vi "Video Processing.vi"() -> ()   [LabVIEW 2014]
uses:
  Global.vi
panel:
  out "Number of Particles before":i32
  out "Processed Image":T1(plugin-control)
  out "Number of Particles after":i32
  out "Original":T1(plugin-control)
  in  "Number of Erosion":i32=30
  out "x-y":u32=48
  out "Read Video":errorcluster
  in  "stop video":bool
  in  "milliseconds to wait":u32
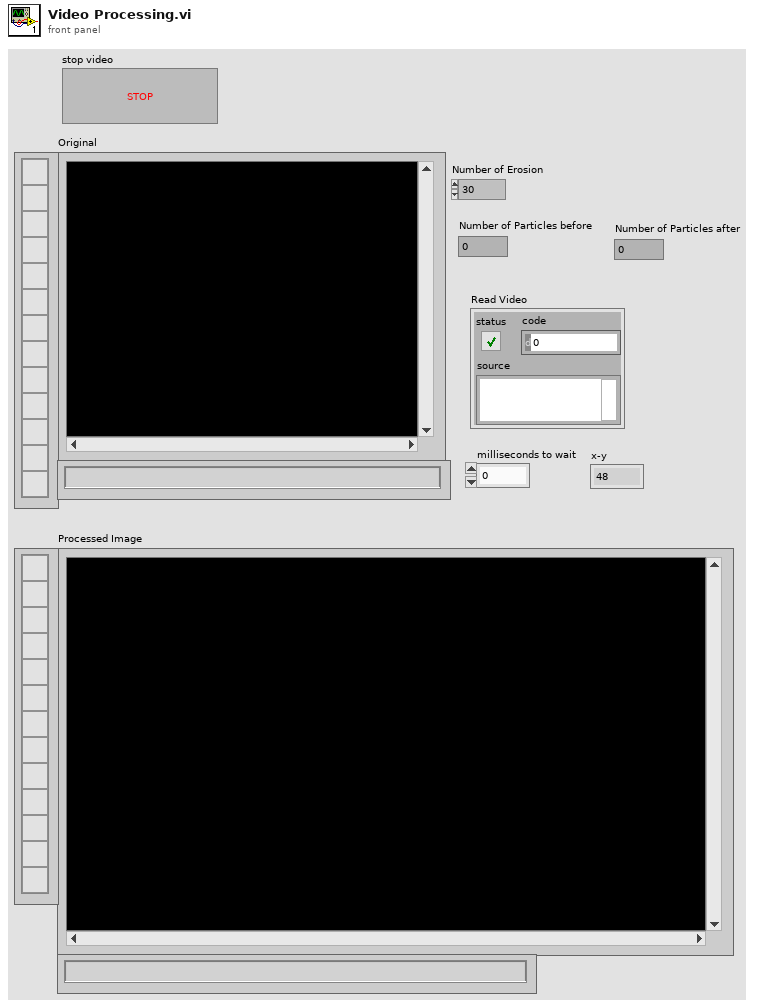
[diagram p1: front panel]
types:
  T1 = typedef "IMAQ Image.ctl" = refnum<image>
  T2 = typedef "Image Type" = u32
  T3 = cluster{"Numeric":dbl, "Numeric":dbl, "Numeric":dbl, "Numeric":dbl}
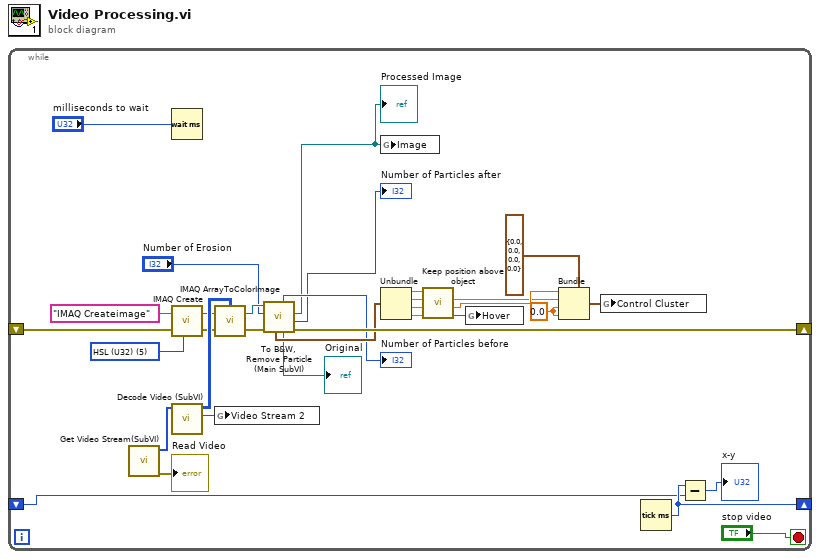
[diagram p0: block diagram]
diagram:
  n1 = while {
    shift-right: [w24] -> _
    shift-left: _ -> [w23]
    shift-right: [w7] -> _
    shift-left: _ -> [w15]
    stop <- "stop video" stop-if-true
    w17 = 0.0
    w30 = T2 5 items=["Grayscale (U8)", "Grayscale (I16)", "Grayscale (SGL)", "Complex (CSG)", "RGB (U32)", "HSL (U32)", "RGB (U64)", "Grayscale (U16)"] ("Image Type")
    n2 = call "Get Video Stream(SubVI).vi"() -> ("error out"=→"Read Video":errorcluster, "ImgData"=w31:u8[])  [unwired: 10 in]
    n3 = Wait (ms)(milliseconds to wait="milliseconds to wait") -> ()  [unwired: 1 out]
    n4 = call "IMAQ Create"("Image Name"="IMAQ Createimage", "Image Type"=w30, "error in (no error)"=w15) -> ("New Image"=w26:T1, "error out"=w25:errorcluster)  [unwired: 2 in]
    n5 = call "Decode Video (SubVI).vi"("ImgData"=w31) -> ("new picture"=w21:picture, "Array"=w27:u32[][])  [unwired: 9 in]
    n6 = call "IMAQ ArrayToColorImage"("Image Pixels (U32)"=w27, "Image"=w26, "error in (no error)"=w25) -> ("Image Out"=w9:T1, "error out"=w8:errorcluster)  [unwired: 2 in]
    n7 = global write "Global.vi" "Video Stream 2"(w21) -> ()
    n8 = call "To B&W, Remove Particle (Main SubVI).vi"("error in (no error)"=w8, "Number of Erosion"="Number of Erosion", "Refnum in"=w9) -> ("error out"=w7:errorcluster, "Number of Particles after"=→"Number of Particles after":i32, "Image Out"=w1:T1, "Original"=→"Original":T1, "Number of Particles before"=→"Number of Particles before":i32, "Cluster"=w5:T3)  [unwired: 3 in]
    "Processed Image" <- w1
    n9 = global write "Global.vi" "Image"(w1) -> ()
    n10 = Unbundle(w5) -> ("Numeric"=w14:dbl, "Numeric"=w13:dbl, "Numeric"=w12:dbl, "Numeric"=w11:dbl)
    n11 = call "Keep position above object.vi"("bottom"=w11, "right"=w12, "top"=w13, "left"=w14) -> ("Hover"=w16:bool, "Roll"=w19:dbl, "Pitch"=w18:dbl)  [unwired: 5 in]
    n12 = global write "Global.vi" "Hover"(w16) -> ()
    n13 = Bundle(cluster=cluster{"Roll":dbl, "Pitch":dbl, dbl, dbl} {"Roll"=0.0, "Pitch"=0.0, 0.0, 0.0}, "Roll"=w19, "Pitch"=w18, w17, w17) -> (w20:cluster{"Roll":dbl, "Pitch":dbl, dbl, dbl})
    n14 = global write "Global.vi" "Control Cluster"(w20) -> ()
    n15 = Tick Count (ms)() -> (millisecond timer value=w24:u32)
    n16 = Subtract(x=w24, y=w23) -> (x-y=→"x-y":u32)
  }
